vi "Brass_3.vi"(0 "Amount":fxp<+,8,0>, 4 "S/R":fxp<+,16,0>, 5 "1/Decay":fxp<+,16,0>, 6 "Sustain":fxp<+,16,0>, 7 "1/Attack":fxp<+,16,0>, 8 "Gate":bool, 9 "LFO":fxp<+/-,8,8>, 10 "M":fxp<+,32,32>, 11 "Trigger":bool) -> (3 "Brass Out":fxp<+/-,8,8>)   [LabVIEW 2015]
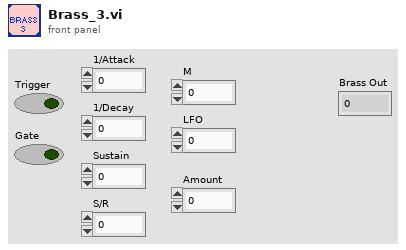
[diagram p1: front panel]
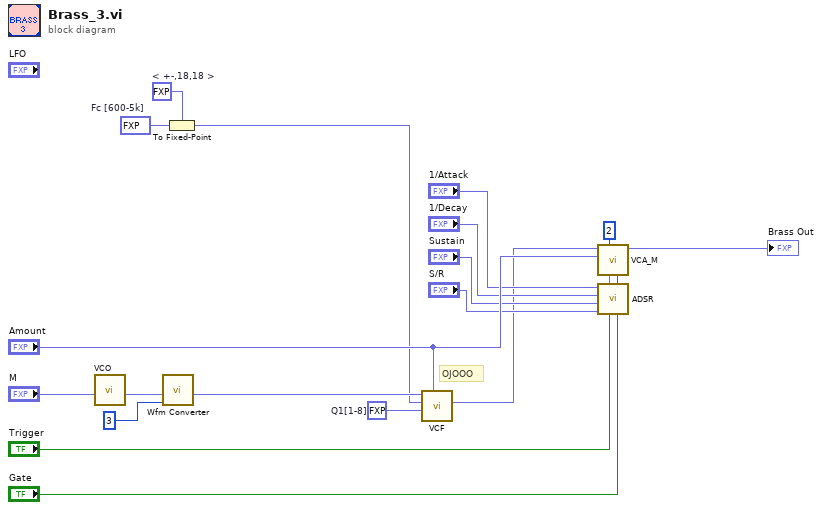
[diagram p0: block diagram]
diagram:
  w9 = fxp<+/-,32,16> 3000.0  # Fc [600-5k]
  w11 = fxp<+/-,18,18> 1.0  # Q1[1-8]
  w10 = fxp<+/-,18,18> 0.0  # < +-,18,18 >
  # "OJOOO"
  n1 = call "VCO.vi"("M"="M") -> ("Sine Sample"=w6:fxp<+/-,8,8>)  [unwired: 10 in]
  n2 = call "Wfm Converter.vi"("Select"=u8 3 ("select"), "Sample In"=w6) -> ("Sample Out"=w8:fxp<+/-,8,8>)  [unwired: 9 in]
  n3 = To Fixed-Point(fixed-point type=w10, number=w9) -> (fixed-point=w1:fxp<+/-,18,18>)
  n4 = call "VCF.vi"("Amount"="Amount", "Q1"=w11, "F1"=w1, "Sample In"=w8) -> ("LP Out"=w4:fxp<+/-,8,8>)  [unwired: 5 in, 2 out]
  n5 = call "ADSR.vi"("Gate"="Gate", "Trigger"="Trigger", "S/R"="S/R", "Sustain"="Sustain", "1/Decay"="1/Decay", "1/Attack"="1/Attack") -> ("Amount?"=w17:bool, "Sample Out"=w16:fxp<+,8,0>)  [unwired: 4 in]
  n6 = call "VCA_M.vi"("Amount?"=w17, "EG"=w16, "Scale"=i8 2, "Amount"="Amount", "Sample In"=w4) -> ("Sample Out"=→"Brass Out":fxp<+/-,8,8>)  [unwired: 6 in]
